vi "Initialize Instrument.vi"(8 "error in (no error)":errorcluster, 10 "Reset":bool, 11 "SA-FSW in":refnum<class "SA-FSW.lvclass">) -> (0 "error out":errorcluster, 3 "SA-FSW out":refnum<class "SA-FSW.lvclass">)   [LabVIEW 2020, in "SA-FSW.lvclass"]
uses:
  SA-FSW.lvclass
  C:/Sandbox/Git_Sandbox/WiSpry Test Framework source code (LV20)/WiSpry Test Framework/Instruments/Instrument.lvclass
  C:/Sandbox/Git_Sandbox/WiSpry Test Framework source code (LV20)/WiSpry Test Framework/Instruments/Spectrum Analyzer/Spectrum Analyzer.lvclass
  Instrument.lvclass/Instrument.ctl
  Spectrum Analyzer.lvclass/Spectrum Analyzer.ctl
  <vilib>/Utility/config.llb/Read Key (Double).vi
  Instrument.lvclass
  <vilib>/Utility/config.llb/NI_LVConfig.lvlib
  Spectrum Analyzer.lvclass
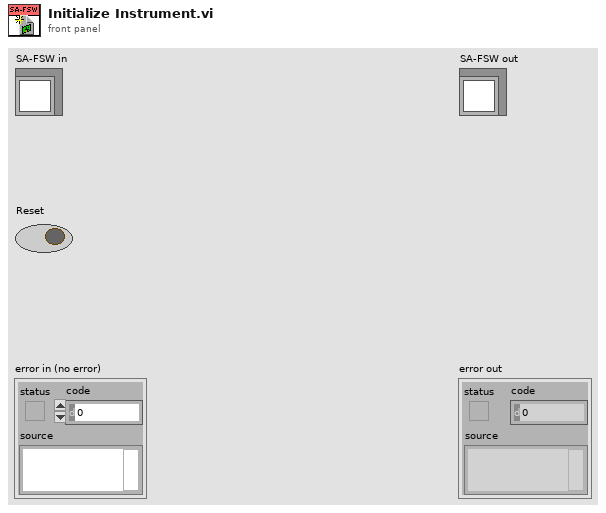
[diagram p1: front panel]
types:
  T1 = typedef "NI_LVConfig.lvlib/Config Data RefNum.ctl" = refnum<k1>
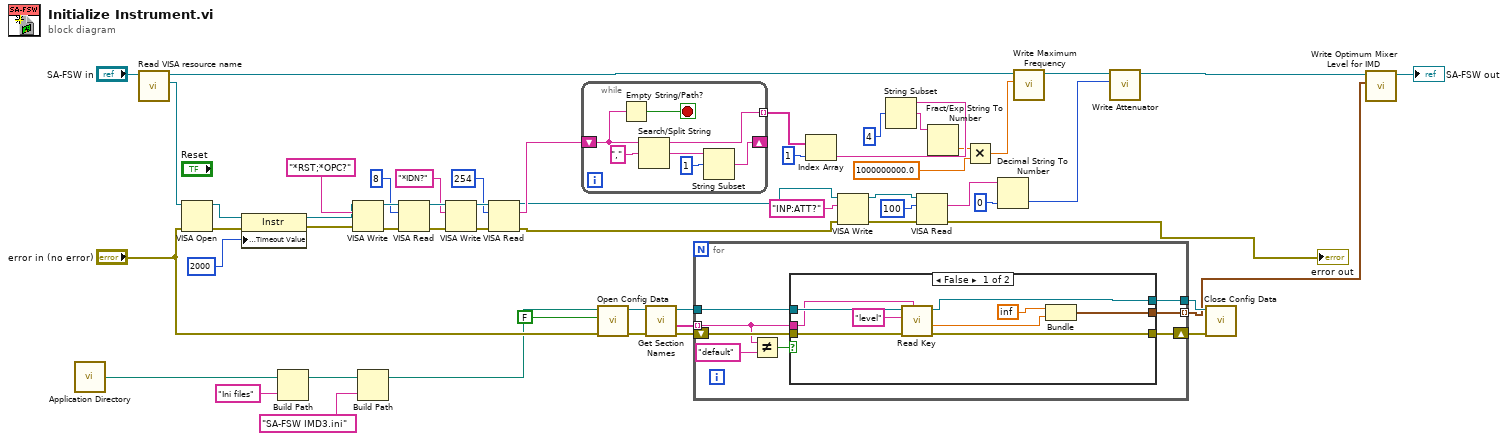
[diagram p0: block diagram]
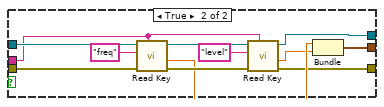
[diagram p2: hidden frame]
diagram:
  n1 = call <vilib>:"Application Directory.vi"() -> ("Application Directory"=w32:path)
  n2 = call "Read VISA resource name.vi"("Instrument in"="SA-FSW in") -> ("VISA resource name"=w54:refnum<visa-resource-name>, "Instrument out"=w34:refnum<class "SA-FSW.lvclass">)  [unwired: 9 in]
  n3 = VISA Open(error in (no error)="error in (no error)", VISA resource name=w54) -> (VISA resource name=w19:refnum<visa-resource-name>, error out=w17:errorcluster)  [unwired: 3 in]
  n4 = property class="Instr"(reference=w19, error in=w17, "General Settings:Timeout Value"=u32 2000) -> (reference out=w18:refnum<visa-resource-name>, error out=w16:errorcluster)
  n5 = Build Path(base path=w32, name or relative path="Ini files") -> (appended path=w31:path)
  n6 = VISA Write(VISA resource name=w18, write buffer="*RST;*OPC?", error in (no error)=w16) -> (VISA resource name out=w51:refnum<visa-resource-name>, error out=w52:errorcluster)  [unwired: 1 out]
  n7 = Build Path(base path=w31, name or relative path="SA-FSW IMD3.ini") -> (appended path=w14:path)
  n8 = VISA Read(VISA resource name=w51, byte count=u32 8, error in (no error)=w52) -> (VISA resource name out=w48:refnum<visa-resource-name>, error out=w49:errorcluster)  [unwired: 2 out]
  n9 = VISA Write(VISA resource name=w48, write buffer="*IDN?", error in (no error)=w49) -> (VISA resource name out=w45:refnum<visa-resource-name>, error out=w46:errorcluster)  [unwired: 1 out]
  n10 = VISA Read(VISA resource name=w45, byte count=u32 254, error in (no error)=w46) -> (VISA resource name out=w6:refnum<visa-resource-name>, read buffer=w43:string, error out=w7:errorcluster)  [unwired: 1 out]
  n11 = while {
    tunnel: [w60] -> w42 mode=indexing
    shift-right: [w57] -> _
    shift-left: w43 -> [w61]
    stop <- w62 stop-if-true
    n12 = Empty String/Path?(string/path=w61) -> (empty?=w62:bool)
    n13 = Search/Split String(string=w61, search string/char (-)=",") -> (substring before match=w60:string, match + rest of string=w59:string)  [unwired: 1 in, 1 out]
    n14 = String Subset(string=w59, offset (0)=1) -> (substring=w57:string)  [unwired: 1 in]
  }
  n15 = call <vilib>:"Open Config Data.vi"("error in (no error)"="error in (no error)", "create file if necessary (T)"=FALSE, "configuration file path"=w14) -> ("error out"=w29:errorcluster, "refnum"=w28:T1)  [unwired: 6 in, 1 out]
  n16 = call <vilib>:"Get Section Names.vi"("error in (no error)"=w29, "refnum"=w28) -> ("error out"=w27:errorcluster, "section names"=w26:string[], "refnum out"=w25:T1)  [unwired: 7 in]
  n17 = for {
    tunnel: w26 -> [w66] mode=indexing
    tunnel: w25 -> [w67]
    shift-right: [w64] -> w24
    shift-left: w27 -> [w68]
    tunnel: [w65] -> w21 mode=indexing
    tunnel: [w63] -> w23
    n18 = Not Equal?(x=w66, y="default") -> (x != y?=w69:bool)
    n19 = case shown="False" w69 {
      tunnel: w68 -> [w79 w91]
      tunnel: w67 -> [w78 w90]
      tunnel: w66 -> [w77 w88]
      tunnel: [w71 w82] -> w65
      tunnel: [w73 w81] -> w64
      tunnel: [w72 w80] -> w63
      frame False {
        n20 = call-poly <vilib>:"Read Key.vi"("section"=w77, "error in (no error)"=w79, "key"="level", "refnum"=w78) -> ("error out"=w73:errorcluster, "value"=w74:dbl, "refnum out"=w72:T1)  [unwired: 4 in, 1 out]
        n21 = Bundle(inf, "value"=w74) -> (w71:cluster{dbl, "value":dbl})  [unwired: 1 in]
      }
      frame True {
        n22 = call-poly <vilib>:"Read Key.vi"("section"=w88, "error in (no error)"=w91, "key"="freq", "refnum"=w90) -> ("error out"=w89:errorcluster, "value"=w84:dbl, "refnum out"=w86:T1)  [unwired: 4 in, 1 out]
        n23 = call-poly <vilib>:"Read Key.vi"("section"=w88, "error in (no error)"=w89, "key"="level", "refnum"=w86) -> ("error out"=w81:errorcluster, "value"=w83:dbl, "refnum out"=w80:T1)  [unwired: 4 in, 1 out]
        n24 = Bundle("value"=w84, "value"=w83) -> (w82:cluster{"value":dbl, "value":dbl})  [unwired: 1 in]
      }
    }
  }
  n25 = Index Array(array=w42, index=1) -> (element=w40:string)
  n26 = VISA Write(VISA resource name=w6, write buffer="INP:ATT?", error in (no error)=w7) -> (VISA resource name out=w10:refnum<visa-resource-name>, error out=w11:errorcluster)  [unwired: 1 out]
  n27 = String Subset(string=w40, offset (0)=4) -> (substring=w38:string)  [unwired: 1 in]
  n28 = VISA Read(VISA resource name=w10, byte count=u32 100, error in (no error)=w11) -> (read buffer=w5:string, error out=→"error out":errorcluster)  [unwired: 2 out]
  n29 = Fract/Exp String To Number(string=w38) -> (number=w37:dbl)  [unwired: 3 in, 1 out]
  n30 = Multiply(x=w37, y=1000000000.0) -> (x*y=w35:dbl)
  n31 = Decimal String To Number(string=w5, default (0L)=u32 0) -> (number=w1:u32)  [unwired: 1 in, 1 out]
  n32 = call "Write Maximum Frequency.vi"("Maximum Frequency"=w35, "Spectrum Analyzer in"=w34) -> ("Spectrum Analyzer out"=w3:refnum<class "SA-FSW.lvclass">)  [unwired: 9 in]
  n33 = call "Write Attenuator.vi"("Attenuator"=w1, "Spectrum Analyzer in"=w3) -> ("Spectrum Analyzer out"=w2:refnum<class "SA-FSW.lvclass">)  [unwired: 9 in]
  n34 = call <vilib>:"Close Config Data.vi"("error in (no error)"=w24, "refnum"=w23) -> ()  [unwired: 8 in, 2 out]
  n35 = call "Write Optimum Mixer Level for IMD.vi"("Optimum Mixer Level for IMD"=w21, "Spectrum Analyzer in"=w2) -> ("Spectrum Analyzer out"=→"SA-FSW out":refnum<class "SA-FSW.lvclass">)  [unwired: 9 in]
